vi "_VISA Read.vi"(8 "error in (no error)":errorcluster, 10 "byte count":u32=1024, 11 "VISA resource name":refnum<visa-resource-name>="GPIB0::23::INSTR") -> (0 "error out":errorcluster, 2 "read buffer":string, 3 "VISA resource name out":refnum<visa-resource-name>)   [LabVIEW 2017, in "SR400.lvlib"]
uses:
  SR400.lvlib
  Global/GPIB Numbers.vi
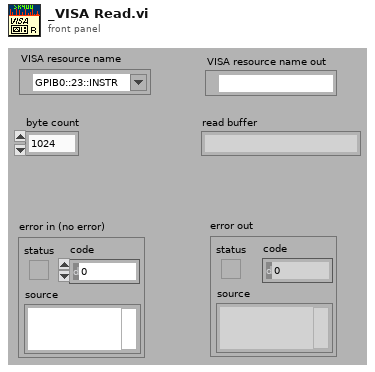
[diagram p1: front panel]
types:
  T1 = typedef "GPIB Type Def.ctl" = cluster{"Name":string, "bus":dbl, "GPIB":dbl, "GPIB as string":string, "byte":i32, "VISA Resource Name":refnum<visa-resource-name>}
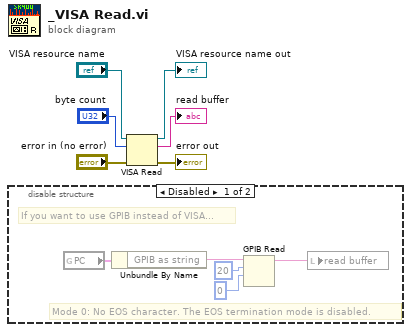
[diagram p0: block diagram]
diagram:
  n1 = disable-structure shown="Disabled" {
    frame Disabled {
      # "Mode 0: No EOS character. The EOS termination mode is disabled."
      # "If you want to use GPIB instead of VISA..."
      n2 = global read "GPIB Numbers.vi" "PC"() -> (w11:T1)
      n3 = Unbundle By Name(w11) -> ("GPIB as string"=w9:string)
      n4 = GPIB Read(0:w9, 1:20 ("byte count"), 2:0) -> (5:w8:string)  [unwired: 1 in, 3 out]
      n5 = local write "read buffer"(w8) -> ()
    }
    frame Enabled {
    }
  }
  n6 = VISA Read(VISA resource name="VISA resource name", byte count="byte count", error in (no error)="error in (no error)") -> (VISA resource name out=→"VISA resource name out":refnum<visa-resource-name>, read buffer=→"read buffer":string, error out=→"error out":errorcluster)  [unwired: 1 out]
